vi "STM_Client_OO.vi"() -> ()   [LabVIEW 2016, in "RemoteControl.STM.lvclass"]
uses:
  RemoteControl.STM.lvclass
  <vilib>/NI/STM/SubVIs/MetaDataElement.ctl
  RemoteControl.STM.lvclass/RemoteControl.STM.ctl
  <userlib>/_OpenG.lib/error/error.llb/Filter Error Codes (Array)__ogtk.vi
  RemoteControl/RemoteControl.lvclass
  <vilib>/NI/STM/NI STM.lvlib
panel:
  in  "milliseconds to wait":u32
  out "time (1 message) (ms)":u32
  out "startup time (ms)":u32
  out "messsages/s":dbl
  in  "remote port":u16=6341
  in  "address":string
  out "Data reponse":variant
  out "time (ms)":u32
  out "Numeric":i32
  out "Data":string
  in  "Stop":bool
  out "Command reponse":string
  out "Command":string
  out "meta data\n(available commands)":T1[](array[typedef])
  out "error out":errorcluster
  # "CLIENT (API)"
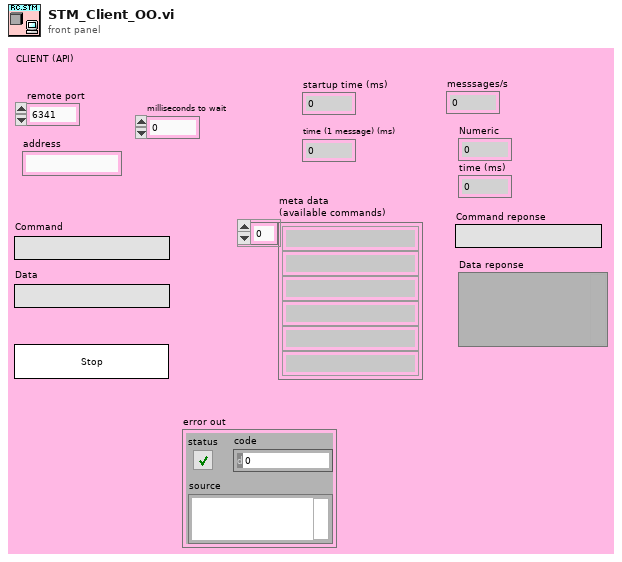
[diagram p1: front panel]
types:
  T1 = typedef "NI STM.lvlib/MetaDataElement.ctl" = string
  T2 = cluster{"Command out":string, "Data out":variant, i32}
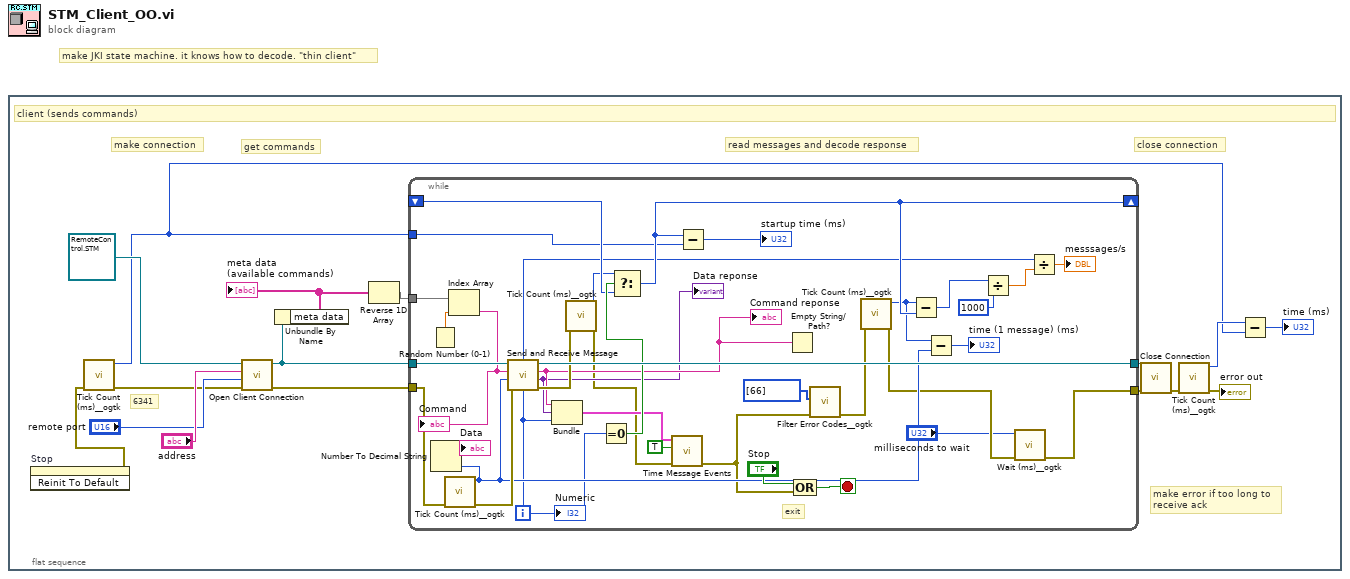
[diagram p0: block diagram]
diagram:
  # "make JKI state machine. it knows how to decode. \"thin client\""
  n1 = flat-sequence {
    frame #0 {
      # "close connection"
      # "read messages and decode response"
      # "get commands"
      # "make connection"
      # "6341"
      # "make error if too long to\nreceive ack"
      # "client (sends commands)"
      n2 = invoke on="Stop" class="Bool" method="Reinit To Default"() -> (error out=w13:errorcluster)  [unwired: 3 in, 2 out]
      n3 = call <userlib>:"Tick Count (ms)__ogtk.vi"("error in (no error)"=w13) -> ("error out"=w6:errorcluster, "millisecond timer value"=w3:u32)  [unwired: 9 in]
      n4 = call-dynamic "Open Client Connection.vi"("error in (no error)"=w6, "Port"="remote port", "address"="address", "RemoteControl.STM in"=refnum<class "RemoteControl.STM.lvclass"> refnum) -> ("error out"=w4:errorcluster, "RemoteControl.STM out"=w9:refnum<class "RemoteControl.STM.lvclass">)  [unwired: 6 in]
      n5 = Unbundle By Name(w9) -> ("meta data"=w2:T1[])
      "meta data\n(available commands)" <- w2
      n6 = Reverse 1D Array(array=w2) -> (reversed array=w1:T1[])
      n7 = while {
        tunnel: [w18] -> w16
        tunnel: [w48] -> w15
        tunnel: w4 -> [w30]
        tunnel: w9 -> [w49]
        tunnel: w3 -> [w37]
        shift-right: [w38] -> _
        shift-left: _ -> [w39]
        tunnel: w1 -> [w36]
        i -> [w24]
        stop <- w52 stop-if-true
        # "exit"
        n8 = Random Number (0-1)() -> (number: 0 to 1=w35:dbl)
        n9 = call <userlib>:"Tick Count (ms)__ogtk.vi"("error in (no error)"=w30) -> ("error out"=w29:errorcluster, "millisecond timer value"=w28:u32)  [unwired: 9 in]
        n10 = Number To Decimal String(number=w28) -> (decimal integer string=→"Data":string)  [unwired: 1 in]
        n11 = Index Array(array=w36, index=w35) -> (element=w34:T1)
        "Command" <- w34
        n12 = call-dynamic "Send and Receive Message.vi"("error in (no error)"=w29, "Data"=w28, "Command"=w34, "RemoteControl in"=w49) -> ("error out"=w42:errorcluster, "Data out"=w25:variant, "Command out"=w26:string, "RemoteControl out"=w48:refnum<class "RemoteControl.STM.lvclass">)  [unwired: 4 in]
        "Command reponse" <- w26
        "Data reponse" <- w25
        n13 = Bundle("Command out"=w26, "Data out"=w25, w24) -> (w23:T2)  [unwired: 1 in]
        n14 = call <userlib>:"Tick Count (ms)__ogtk.vi"("error in (no error)"=w42) -> ("error out"=w21:errorcluster, "millisecond timer value"=w32:u32)  [unwired: 9 in]
        n15 = Equal To 0?(x=w24) -> (x = 0?=w40:bool)
        n16 = Select(t=w32, s=w40, f=w39) -> (s? t:f=w38:u32)
        n17 = call "Time Message Events.vi"("error in (no error)"=w21, "Debug Mode"=TRUE, "Message in"=w23) -> ("error out"=w20:errorcluster)  [unwired: 6 in, 2 out]
        n18 = Subtract(x=w38, y=w37) -> (x-y=→"startup time (ms)":u32)
        n19 = Empty String/Path?(string/path=w26) -> ()  [unwired: 1 out]
        n20 = Compound Arithmetic op=OR("Stop", w20) -> (w52:bool)
        n21 = call-poly <userlib>:"Filter Error Codes__ogtk.vi"("Error In"=w20, "Error Codes to Filter"=i32[] [66]) -> ("Error Out"=w47:errorcluster)  [unwired: 7 in, 2 out]
        n22 = call <userlib>:"Tick Count (ms)__ogtk.vi"("error in (no error)"=w47) -> ("error out"=w19:errorcluster, "millisecond timer value"=w33:u32)  [unwired: 9 in]
        n23 = Subtract(x=w33, y=w38) -> (x-y=w44:u32)
        n24 = Subtract(x=w33, y=w28) -> (x-y=→"time (1 message) (ms)":u32)
        n25 = Divide(x=w44, y=u32 1000) -> (x/y=w46:dbl)
        n26 = call <userlib>:"Wait (ms)__ogtk.vi"("error in (no error)"=w19, "milliseconds to wait"="milliseconds to wait") -> ("error out"=w18:errorcluster)  [unwired: 8 in, 1 out]
        n27 = Divide(x=w24, y=w46) -> (x/y=→"messsages/s":dbl)
        "Numeric" <- w24
      }
      n28 = call-dynamic "Close Connection.vi"("error in (no error)"=w16, "RemoteControl.STM in"=w15) -> ("error out"=w14:errorcluster)  [unwired: 8 in, 1 out]
      n29 = call <userlib>:"Tick Count (ms)__ogtk.vi"("error in (no error)"=w14) -> ("error out"=→"error out":errorcluster, "millisecond timer value"=w11:u32)  [unwired: 9 in]
      n30 = Subtract(x=w11, y=w3) -> (x-y=→"time (ms)":u32)
    }
  }
